vi "PS-RA03B FPGA.vi"() -> ()   [LabVIEW 2011]
uses:
  <vilib>/rvi/eio/common/nirviEmuTemplateMethod_errors.vi
  <vilib>/eio/EIONode/EIONode.xnode
  <vilib>/eio/EIOMethodNode/EIOMethodNode.xnode
  Filter VIs.lvlib
panel:
  out "Timestamp":u32 caption="Tick Count(Ticks)"
  out "Mod5/AI0":fxp<+/-,20,5> format="%.17g"
  out "Mod5/AI2":fxp<+/-,20,5> format="%.17g"
  out "Mod5/AI3":fxp<+/-,20,5> format="%.17g"
  out "Mod1/AI0":fxp<+/-,20,5> format="%.17g"
  out "Mod1/AI1":fxp<+/-,20,5> format="%.17g"
  out "Mod1/AI2":fxp<+/-,20,5> format="%.17g"
  out "Mod1/AI3":fxp<+/-,20,5> format="%.17g"
  out "Mod5/AI1":fxp<+/-,20,5> format="%.17g"
  out "period":u32
  out "delay":u32
  out "dperiod":u32
  out "ACH06-Setpoint":fxp<+/-,20,5>
  out "ALV06B-Setpoint":fxp<+/-,20,5>
  out "ACH05B-Setpoint":fxp<+/-,20,5>
  out "ALV06A-Setpoint":fxp<+/-,20,5>
  out "ACV07A-Setpoint":fxp<+/-,20,5>
  out "ACH07A-Setpoint":fxp<+/-,20,5>
  out "ACV05B-Setpoint":fxp<+/-,20,5>
  out "RRA03B-Setpoint":fxp<+/-,20,5>
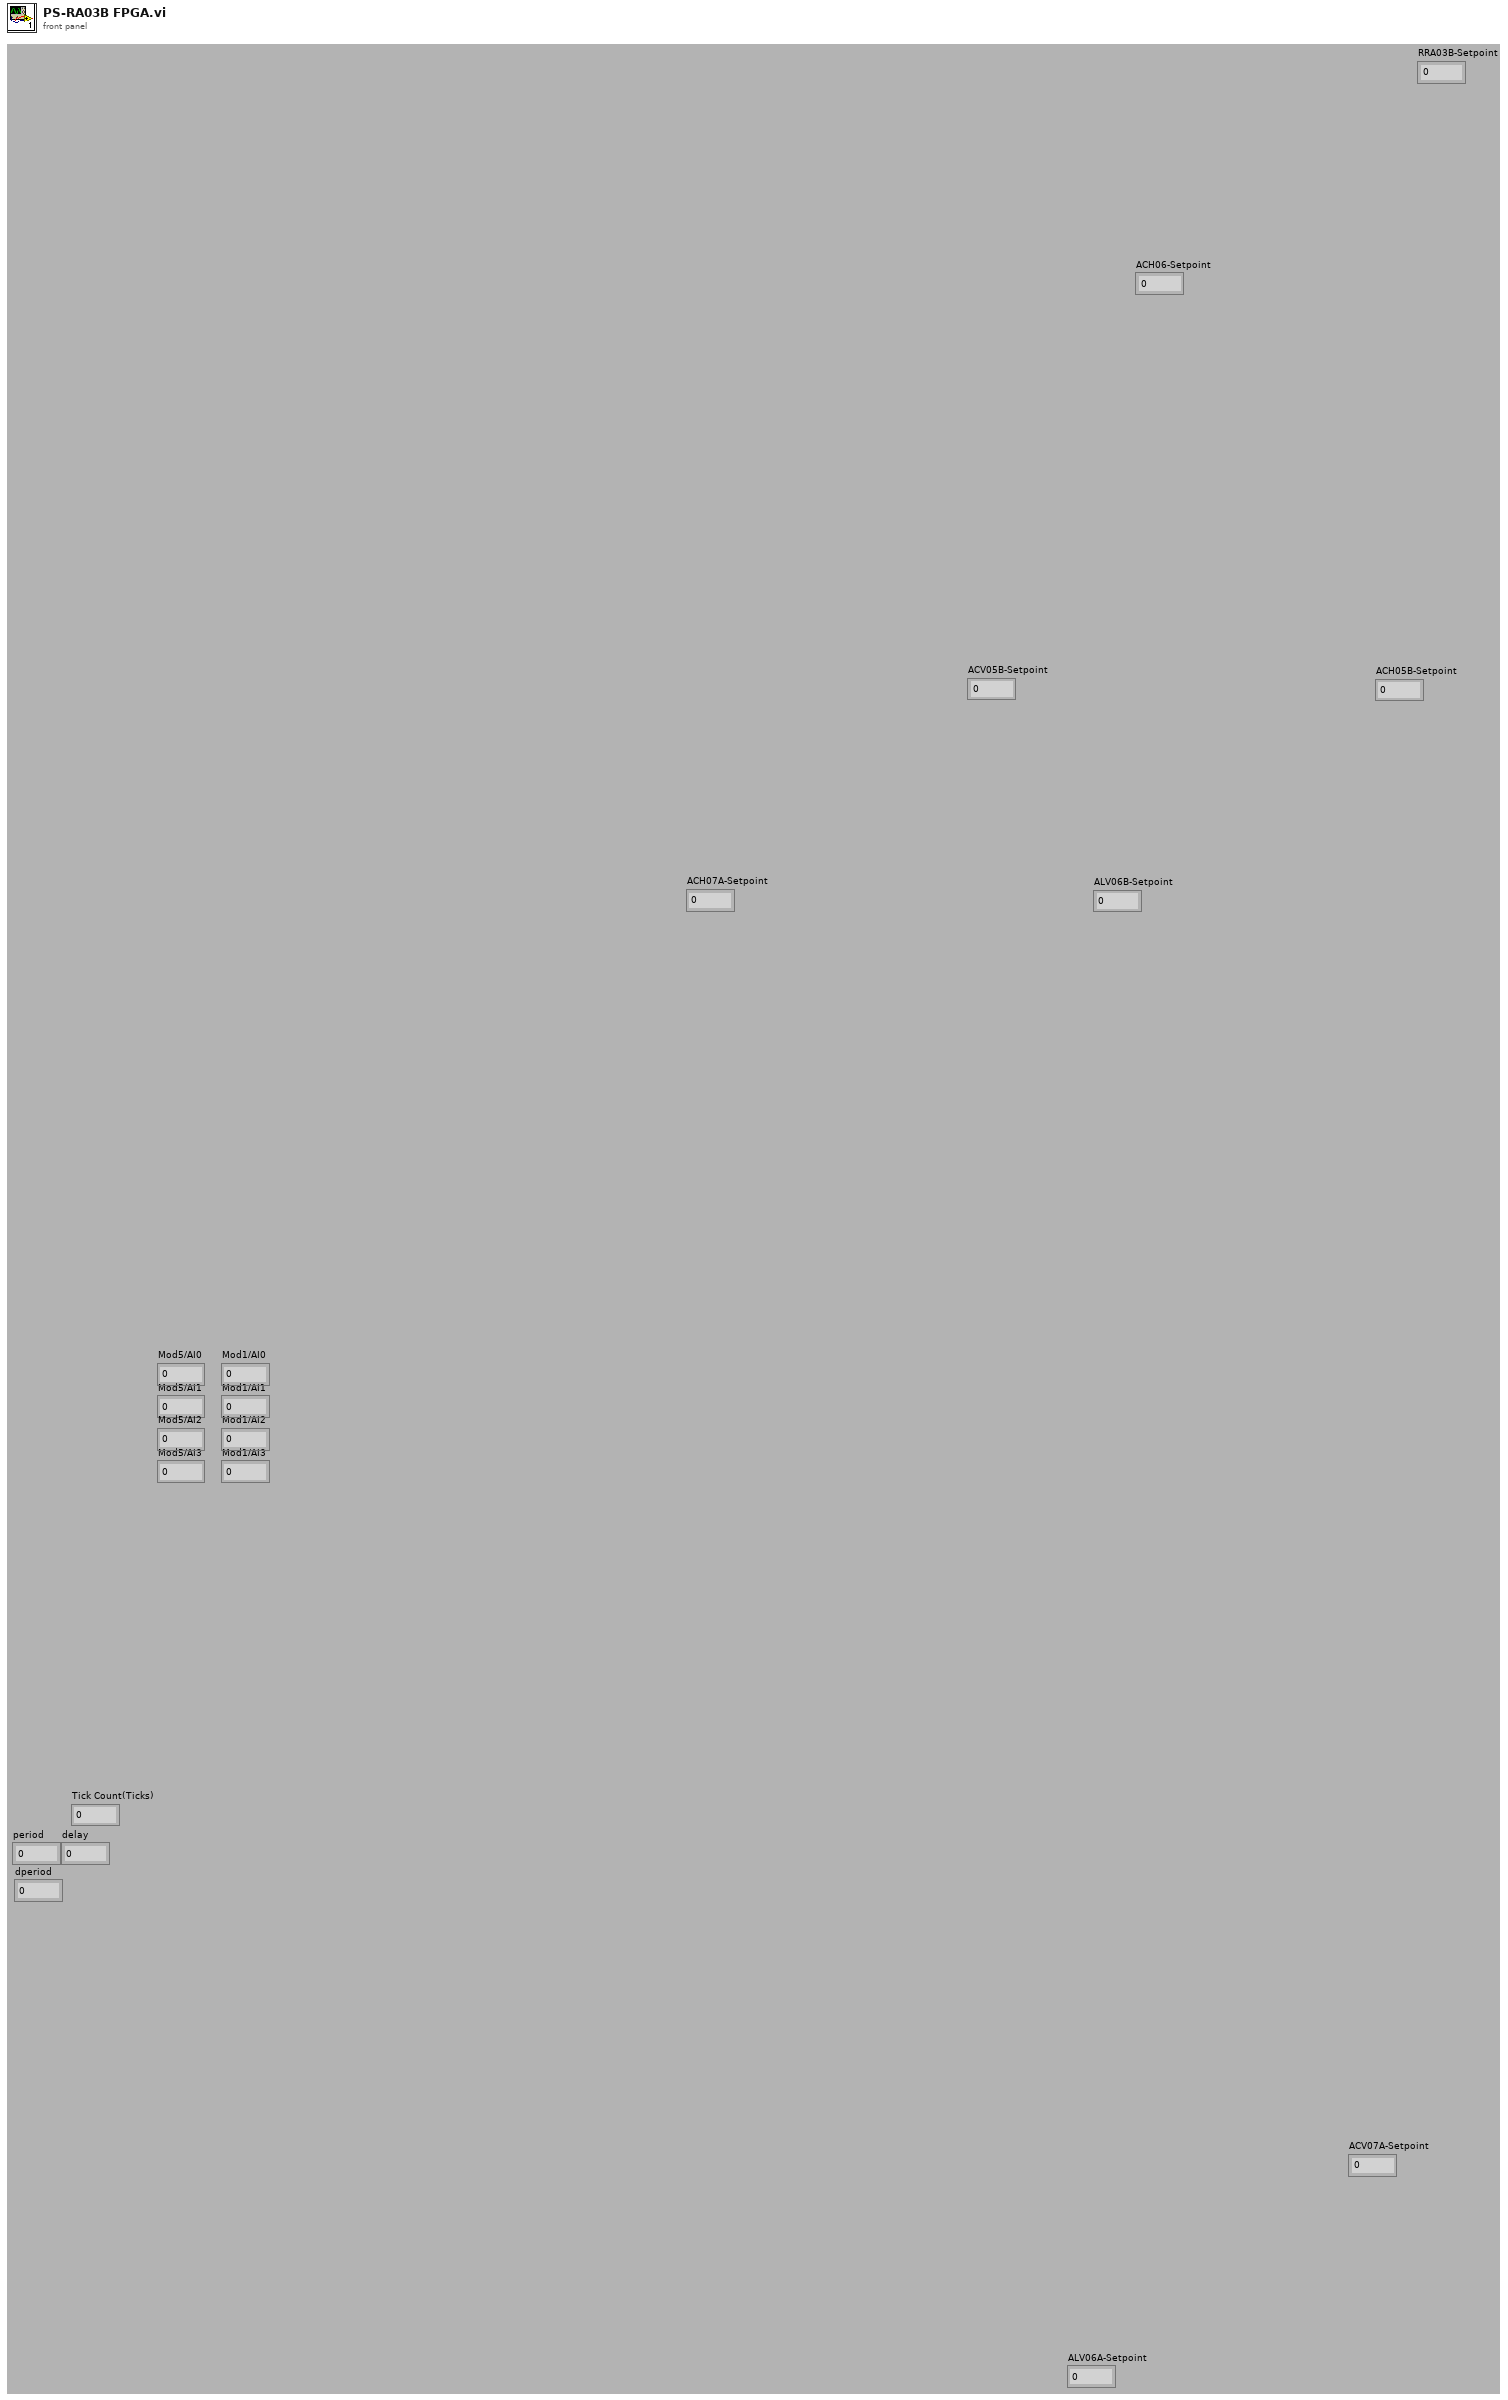
[diagram p1: front panel]
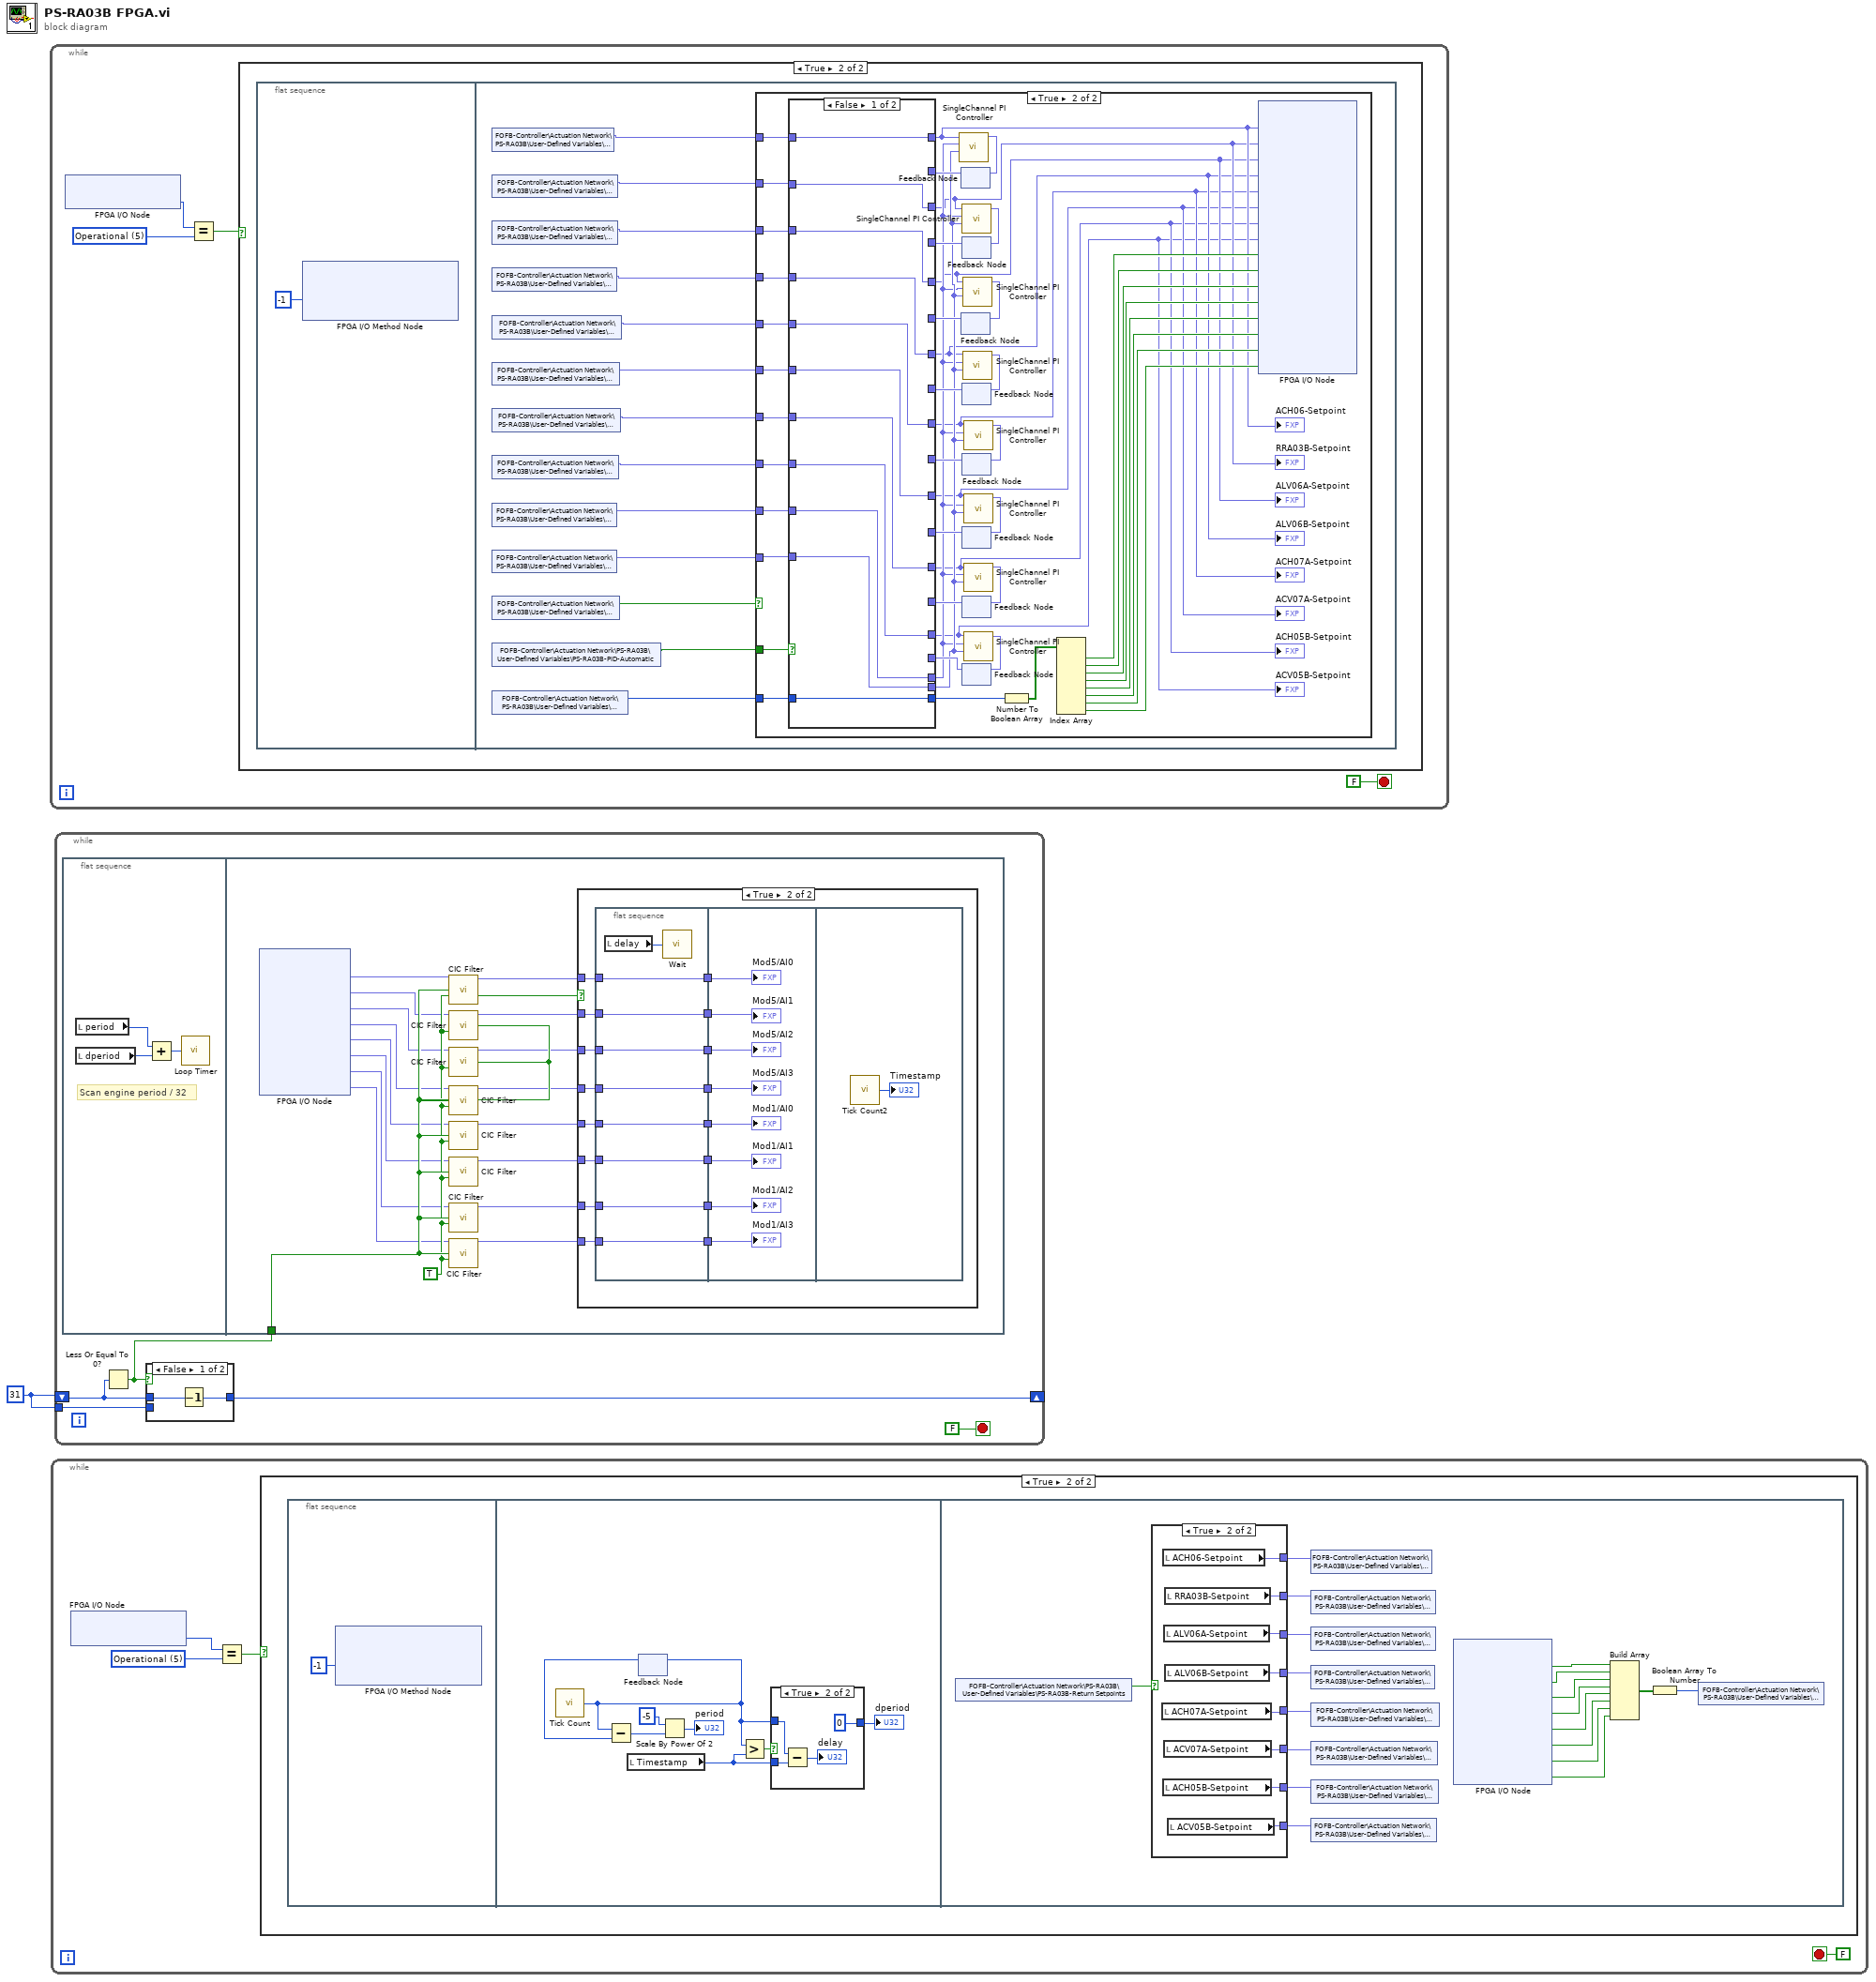
[diagram p0: block diagram]
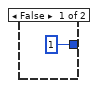
[diagram p5: hidden frame]
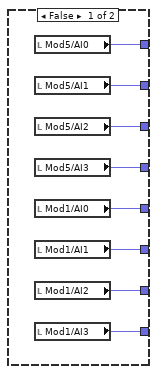
[diagram p6: hidden frame]
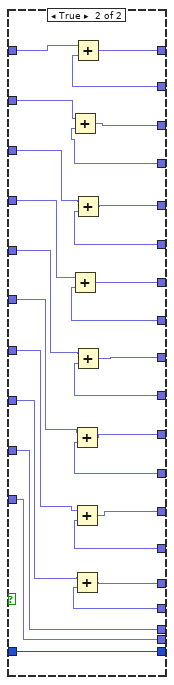
[diagram p9: hidden frame]
diagram:
  w1 = 31
  n1 = while {
    stop <- FALSE stop-if-true
    w4 = u8 5 items=["Init"=1, "PreOp"=2, "Bootstrap"=3, "SafeOp"=4, "Operational"=5]
    n2 = xnode "FPGA I/O Node"() -> ("EtherCAT State"=w3:u8)  [unwired: 1 in, 1 out]
    n3 = Equal?(x=w3, y=w4) -> (x = y?=w2:bool)
    n4 = case shown="True" w2 {
      frame False {
      }
      frame True {
        n5 = flat-sequence {
          frame #0 {
            n6 = xnode "FPGA I/O Method Node"("Timeout"=-1) -> ()  [unwired: 1 in, 2 out]
          }
          frame #1 {
            n7 = shared-variable "FOFB-Controller\\Actuation Network\\PS-RA03B\\User-Defined Variables\\ACH06-Setpoint"() -> (w19:fxp<+/-,20,5>)  [unwired: 1 in, 1 out]
            n8 = shared-variable "FOFB-Controller\\Actuation Network\\PS-RA03B\\User-Defined Variables\\RRA03B-Setpoint"() -> (w18:fxp<+/-,20,5>)  [unwired: 1 in, 1 out]
            n9 = shared-variable "FOFB-Controller\\Actuation Network\\PS-RA03B\\User-Defined Variables\\ALV06A-Setpoint"() -> (w17:fxp<+/-,20,5>)  [unwired: 1 in, 1 out]
            n10 = shared-variable "FOFB-Controller\\Actuation Network\\PS-RA03B\\User-Defined Variables\\ALV06B-Setpoint"() -> (w16:fxp<+/-,20,5>)  [unwired: 1 in, 1 out]
            n11 = shared-variable "FOFB-Controller\\Actuation Network\\PS-RA03B\\User-Defined Variables\\ACH07A-Setpoint"() -> (w15:fxp<+/-,20,5>)  [unwired: 1 in, 1 out]
            n12 = shared-variable "FOFB-Controller\\Actuation Network\\PS-RA03B\\User-Defined Variables\\ACV07A-Setpoint"() -> (w14:fxp<+/-,20,5>)  [unwired: 1 in, 1 out]
            n13 = shared-variable "FOFB-Controller\\Actuation Network\\PS-RA03B\\User-Defined Variables\\ACH05B-Setpoint"() -> (w13:fxp<+/-,20,5>)  [unwired: 1 in, 1 out]
            n14 = shared-variable "FOFB-Controller\\Actuation Network\\PS-RA03B\\User-Defined Variables\\ACV05B-Setpoint"() -> (w12:fxp<+/-,20,5>)  [unwired: 1 in, 1 out]
            n15 = shared-variable "FOFB-Controller\\Actuation Network\\PS-RA03B\\User-Defined Variables\\PS-RA03B-PID-I1"() -> (w11:fxp<+/-,18,1>)  [unwired: 1 in, 1 out]
            n16 = shared-variable "FOFB-Controller\\Actuation Network\\PS-RA03B\\User-Defined Variables\\PS-RA03B-PID-I2"() -> (w10:fxp<+/-,18,2>)  [unwired: 1 in, 1 out]
            n17 = shared-variable "FOFB-Controller\\Actuation Network\\PS-RA03B\\User-Defined Variables\\PS-RA03B-Enable"() -> (w7:bool)  [unwired: 1 in, 1 out]
            n18 = shared-variable "FOFB-Controller\\Actuation Network\\PS-RA03B\\User-Defined Variables\\PS-RA03B-PID-Automatic"() -> (w9:bool)  [unwired: 1 in, 1 out]
            n19 = shared-variable "FOFB-Controller\\Actuation Network\\PS-RA03B\\User-Defined Variables\\PS-RA03B-ON-OFF"() -> (w8:u8)  [unwired: 1 in, 1 out]
            n20 = case shown="True" w7 {
              tunnel: w19 -> [_ w39]
              tunnel: w18 -> [_ w38]
              tunnel: w17 -> [_ w37]
              tunnel: w16 -> [_ w36]
              tunnel: w15 -> [_ w35]
              tunnel: w14 -> [_ w34]
              tunnel: w13 -> [_ w33]
              tunnel: w12 -> [_ w32]
              tunnel: w11 -> [_ w31]
              tunnel: w10 -> [_ w30]
              tunnel: w9 -> [_ w29]
              tunnel: w8 -> [_ w28]
              frame False {
              }
              frame True {
                n21 = feedback #1() -> (w65:fxp<+/-,20,5>)  [unwired: 1 in]
                n22 = feedback #2() -> (w63:fxp<+/-,20,5>)  [unwired: 1 in]
                n23 = feedback #3() -> (w64:fxp<+/-,20,5>)  [unwired: 1 in]
                n24 = feedback #4() -> (w62:fxp<+/-,20,5>)  [unwired: 1 in]
                n25 = feedback #5() -> (w61:fxp<+/-,20,5>)  [unwired: 1 in]
                n26 = feedback #6() -> (w60:fxp<+/-,20,5>)  [unwired: 1 in]
                n27 = feedback #7() -> (w59:fxp<+/-,20,5>)  [unwired: 1 in]
                n28 = feedback #8() -> (w58:fxp<+/-,20,5>)  [unwired: 1 in]
                n29 = case shown="False" w29 {
                  tunnel: w28 -> [w78 w105]
                  tunnel: [w78 w105] -> w66
                  tunnel: [w77 w102] -> w27
                  tunnel: w30 -> [w68 w104]
                  tunnel: [w68 w104] -> w49
                  tunnel: w31 -> [w69 w103]
                  tunnel: [w69 w103] -> w48
                  tunnel: [w76 w97] -> w26
                  tunnel: [w75 w94] -> w25
                  tunnel: [w74 w93] -> w24
                  tunnel: [w73 w92] -> w23
                  tunnel: [w72 w91] -> w22
                  tunnel: [w71 w90] -> w21
                  tunnel: [w70 w89] -> w20
                  tunnel: w65 -> [_ w101]
                  tunnel: w39 -> [w77 w100]
                  tunnel: w64 -> [_ w98]
                  tunnel: w63 -> [_ w95]
                  tunnel: w62 -> [_ w79]
                  tunnel: w61 -> [_ w83]
                  tunnel: w60 -> [_ w86]
                  tunnel: w59 -> [_ w87]
                  tunnel: w58 -> [_ w81]
                  tunnel: w32 -> [w70 w82]
                  tunnel: w33 -> [w71 w88]
                  tunnel: w34 -> [w72 w85]
                  tunnel: w35 -> [w73 w84]
                  tunnel: w36 -> [w74 w80]
                  tunnel: w37 -> [w75 w96]
                  tunnel: w38 -> [w76 w99]
                  frame False {
                  }
                  frame True {
                    n30 = Add(x=w99, y=w98) -> (x+y=w97:fxp<+/-,20,5>)
                    n31 = Add(x=w80, y=w79) -> (x+y=w93:fxp<+/-,20,5>)
                    n32 = Add(x=w85, y=w86) -> (x+y=w91:fxp<+/-,20,5>)
                    n33 = Add(x=w88, y=w87) -> (x+y=w90:fxp<+/-,20,5>)
                    n34 = Add(x=w82, y=w81) -> (x+y=w89:fxp<+/-,20,5>)
                    n35 = Add(x=w100, y=w101) -> (x+y=w102:fxp<+/-,20,5>)
                    n36 = Add(x=w96, y=w95) -> (x+y=w94:fxp<+/-,20,5>)
                    n37 = Add(x=w84, y=w83) -> (x+y=w92:fxp<+/-,20,5>)
                  }
                }
                "ACH06-Setpoint" <- w27
                "ALV06B-Setpoint" <- w24
                "ACH05B-Setpoint" <- w21
                "ALV06A-Setpoint" <- w25
                "ACV07A-Setpoint" <- w22
                "ACH07A-Setpoint" <- w23
                "ACV05B-Setpoint" <- w20
                "RRA03B-Setpoint" <- w26
                n38 = call "SingleChannel PI Controller.vi"("Integral Coefficient a[k]"=w49, "Integral Coefficient b[k]"=w48, "input data"=w27) -> ("output data"=w57:fxp<+/-,20,5>)  [unwired: 8 in]
                n39 = feedback-in #1(w57) -> ()
                n40 = call "SingleChannel PI Controller.vi"("Integral Coefficient a[k]"=w49, "Integral Coefficient b[k]"=w48, "input data"=w26) -> ("output data"=w56:fxp<+/-,20,5>)  [unwired: 8 in]
                n41 = feedback-in #3(w56) -> ()
                n42 = call "SingleChannel PI Controller.vi"("Integral Coefficient a[k]"=w49, "Integral Coefficient b[k]"=w48, "input data"=w25) -> ("output data"=w55:fxp<+/-,20,5>)  [unwired: 8 in]
                n43 = feedback-in #2(w55) -> ()
                n44 = call "SingleChannel PI Controller.vi"("Integral Coefficient a[k]"=w49, "Integral Coefficient b[k]"=w48, "input data"=w24) -> ("output data"=w54:fxp<+/-,20,5>)  [unwired: 8 in]
                n45 = feedback-in #4(w54) -> ()
                n46 = call "SingleChannel PI Controller.vi"("Integral Coefficient a[k]"=w49, "Integral Coefficient b[k]"=w48, "input data"=w23) -> ("output data"=w53:fxp<+/-,20,5>)  [unwired: 8 in]
                n47 = feedback-in #5(w53) -> ()
                n48 = call "SingleChannel PI Controller.vi"("Integral Coefficient a[k]"=w49, "Integral Coefficient b[k]"=w48, "input data"=w22) -> ("output data"=w52:fxp<+/-,20,5>)  [unwired: 8 in]
                n49 = feedback-in #6(w52) -> ()
                n50 = call "SingleChannel PI Controller.vi"("Integral Coefficient a[k]"=w49, "Integral Coefficient b[k]"=w48, "input data"=w21) -> ("output data"=w51:fxp<+/-,20,5>)  [unwired: 8 in]
                n51 = feedback-in #7(w51) -> ()
                n52 = call "SingleChannel PI Controller.vi"("Integral Coefficient a[k]"=w49, "Integral Coefficient b[k]"=w48, "input data"=w20) -> ("output data"=w50:fxp<+/-,20,5>)  [unwired: 8 in]
                n53 = feedback-in #8(w50) -> ()
                n54 = Number To Boolean Array(number=w66) -> (Boolean array=w67:bool[])
                n55 = Index Array(array=w67) -> (element #1=w47:bool, element #2=w46:bool, element #3=w45:bool, element #4=w44:bool, element #5=w43:bool, element #6=w42:bool, element #7=w41:bool, element #8=w40:bool)  [unwired: 8 in]
                n56 = xnode "FPGA I/O Node"("Mod6/AO0"=w27, "Mod6/AO1"=w26, "Mod6/AO2"=w25, "Mod6/AO3"=w24, "Mod2/AO0"=w23, "Mod2/AO1"=w22, "Mod2/AO2"=w21, "Mod2/AO3"=w20, "Mod4/DIO6"=w47, "Mod4/DIO7"=w46, "Mod4/DIO4"=w45, "Mod4/DIO5"=w44, "Mod4/DIO2"=w43, "Mod4/DIO3"=w42, "Mod4/DIO0"=w41, "Mod4/DIO1"=w40) -> ()  [unwired: 16 in, 16 out]
              }
            }
          }
        }
      }
    }
  }
  n57 = while {
    stop <- FALSE stop-if-true
    w108 = u8 5 items=["Init"=1, "PreOp"=2, "Bootstrap"=3, "SafeOp"=4, "Operational"=5]
    n58 = xnode "FPGA I/O Node"() -> ("EtherCAT State"=w107:u8)  [unwired: 1 in, 1 out]
    n59 = Equal?(x=w107, y=w108) -> (x = y?=w106:bool)
    n60 = case shown="True" w106 {
      frame False {
      }
      frame True {
        n61 = flat-sequence {
          frame #0 {
            n62 = xnode "FPGA I/O Method Node"("Timeout"=-1) -> ()  [unwired: 1 in, 2 out]
          }
          frame #1 {
            n63 = call "Tick Count"() -> ("Tick Count(Ticks)"=w112:u32)
            n64 = local read "Timestamp"() -> (w114:u32)
            n65 = feedback #9() -> (w111:u32)  [unwired: 1 in]
            n66 = Subtract(x=w112, y=w111) -> (x-y=w117:u32)
            n67 = feedback-in #9(w112) -> ()
            n68 = Scale By Power Of 2(n=i8 -5, x=w117) -> (x*2^n=→"period":u32)
            n69 = Greater?(x=w112, y=w114) -> (0:w115:bool)
            n70 = case shown="True" w115 {
              tunnel: w112 -> [_ w123]
              tunnel: w114 -> [_ w122]
              tunnel: [u32 1 ("dt 2") u32 0 ("dt 2")] -> w113
              frame False {
              }
              frame True {
                n71 = Subtract(x=w123, y=w122) -> (x-y=→"delay":u32)
              }
            }
            "dperiod" <- w113
          }
          frame #2 {
            n72 = shared-variable "FOFB-Controller\\Actuation Network\\PS-RA03B\\User-Defined Variables\\PS-RA03B-Return Setpoints"() -> (w126:bool)  [unwired: 1 in, 1 out]
            n73 = case shown="True" w126 {
              tunnel: [w150 w158] -> w133
              tunnel: [w149 w157] -> w132
              tunnel: [w148 w155] -> w131
              tunnel: [w147 w156] -> w130
              tunnel: [w146 w154] -> w129
              tunnel: [w145 w153] -> w128
              tunnel: [w144 w152] -> w127
              tunnel: [w143 w151] -> w125
              frame False {
                n74 = local read "Mod5/AI0"() -> (w150:fxp<+/-,20,5>)
                n75 = local read "Mod5/AI1"() -> (w149:fxp<+/-,20,5>)
                n76 = local read "Mod5/AI2"() -> (w148:fxp<+/-,20,5>)
                n77 = local read "Mod5/AI3"() -> (w147:fxp<+/-,20,5>)
                n78 = local read "Mod1/AI0"() -> (w146:fxp<+/-,20,5>)
                n79 = local read "Mod1/AI1"() -> (w145:fxp<+/-,20,5>)
                n80 = local read "Mod1/AI2"() -> (w144:fxp<+/-,20,5>)
                n81 = local read "Mod1/AI3"() -> (w143:fxp<+/-,20,5>)
              }
              frame True {
                n82 = local read "ACH07A-Setpoint"() -> (w154:fxp<+/-,20,5>)
                n83 = local read "ACH06-Setpoint"() -> (w158:fxp<+/-,20,5>)
                n84 = local read "ACH05B-Setpoint"() -> (w152:fxp<+/-,20,5>)
                n85 = local read "ALV06A-Setpoint"() -> (w155:fxp<+/-,20,5>)
                n86 = local read "ACV07A-Setpoint"() -> (w153:fxp<+/-,20,5>)
                n87 = local read "RRA03B-Setpoint"() -> (w157:fxp<+/-,20,5>)
                n88 = local read "ALV06B-Setpoint"() -> (w156:fxp<+/-,20,5>)
                n89 = local read "ACV05B-Setpoint"() -> (w151:fxp<+/-,20,5>)
              }
            }
            n90 = shared-variable "FOFB-Controller\\Actuation Network\\PS-RA03B\\User-Defined Variables\\ACH06-Reading"(w133) -> ()  [unwired: 1 in, 1 out]
            n91 = shared-variable "FOFB-Controller\\Actuation Network\\PS-RA03B\\User-Defined Variables\\RRA03B-Reading"(w132) -> ()  [unwired: 1 in, 1 out]
            n92 = shared-variable "FOFB-Controller\\Actuation Network\\PS-RA03B\\User-Defined Variables\\ALV06A-Reading"(w131) -> ()  [unwired: 1 in, 1 out]
            n93 = shared-variable "FOFB-Controller\\Actuation Network\\PS-RA03B\\User-Defined Variables\\ALV06B-Reading"(w130) -> ()  [unwired: 1 in, 1 out]
            n94 = shared-variable "FOFB-Controller\\Actuation Network\\PS-RA03B\\User-Defined Variables\\ACH07A-Reading"(w129) -> ()  [unwired: 1 in, 1 out]
            n95 = shared-variable "FOFB-Controller\\Actuation Network\\PS-RA03B\\User-Defined Variables\\ACV07A-Reading"(w128) -> ()  [unwired: 1 in, 1 out]
            n96 = shared-variable "FOFB-Controller\\Actuation Network\\PS-RA03B\\User-Defined Variables\\ACH05B-Reading"(w127) -> ()  [unwired: 1 in, 1 out]
            n97 = shared-variable "FOFB-Controller\\Actuation Network\\PS-RA03B\\User-Defined Variables\\ACV05B-Reading"(w125) -> ()  [unwired: 1 in, 1 out]
            n98 = xnode "FPGA I/O Node"() -> ("Mod3/DIO6"=w141:bool, "Mod3/DIO7"=w140:bool, "Mod3/DIO4"=w139:bool, "Mod3/DIO5"=w138:bool, "Mod3/DIO2"=w137:bool, "Mod3/DIO3"=w136:bool, "Mod3/DIO0"=w135:bool, "Mod3/DIO1"=w134:bool)  [unwired: 8 in, 8 out]
            n99 = Build Array(w141, w140, w139, w138, w137, w136, w135, w134) -> (w142:bool[])
            n100 = Boolean Array To Number(Boolean array=w142) -> (number=w124:u8)
            n101 = shared-variable "FOFB-Controller\\Actuation Network\\PS-RA03B\\User-Defined Variables\\PS-RA03B-Status"(w124) -> ()  [unwired: 1 in, 1 out]
          }
        }
      }
    }
  }
  n102 = while {
    shift-right: [w162] -> _
    shift-left: w1 -> [w161]
    tunnel: w1 -> [w159]
    stop <- FALSE stop-if-true
    n103 = flat-sequence {
      tunnel: w160 -> [w188]
      frame #0 {
        # "Scan engine period / 32"
        n104 = local read "period"() -> (w169:u32)
        n105 = local read "dperiod"() -> (w168:u32)
        n106 = Add(x=w169, y=w168) -> (x+y=w167:u32)
        n107 = call "Loop Timer"("Count(Ticks)"=w167) -> ()  [unwired: 1 out]
      }
      frame #1 {
        w187 = TRUE ("input valid")
        n108 = xnode "FPGA I/O Node"() -> ("Mod5/AI0"=w177:fxp<+/-,20,5>, "Mod5/AI1"=w176:fxp<+/-,20,5>, "Mod5/AI2"=w175:fxp<+/-,20,5>, "Mod5/AI3"=w174:fxp<+/-,20,5>, "Mod1/AI0"=w173:fxp<+/-,20,5>, "Mod1/AI1"=w172:fxp<+/-,20,5>, "Mod1/AI2"=w171:fxp<+/-,20,5>, "Mod1/AI3"=w170:fxp<+/-,20,5>)  [unwired: 8 in, 8 out]
        n109 = call "CIC Filter.vi"("input data"=w177, "sample"=w188, "input valid"=w187) -> ("output data"=w185:fxp<+/-,20,5>, "output valid"=w186:bool)  [unwired: 10 in, 1 out]
        n110 = call "CIC Filter.vi"("input data"=w176, "sample"=w188, "input valid"=w187) -> ("output data"=w184:fxp<+/-,20,5>)  [unwired: 10 in, 2 out]
        n111 = call "CIC Filter.vi"("input data"=w175, "sample"=w188, "input valid"=w187) -> ("output data"=w183:fxp<+/-,20,5>)  [unwired: 10 in, 2 out]
        n112 = call "CIC Filter.vi"("input data"=w174, "sample"=w188, "input valid"=w187) -> ("output data"=w182:fxp<+/-,20,5>)  [unwired: 10 in, 2 out]
        n113 = call "CIC Filter.vi"("input data"=w173, "sample"=w188, "input valid"=w187) -> ("output data"=w181:fxp<+/-,20,5>)  [unwired: 10 in, 2 out]
        n114 = call "CIC Filter.vi"("input data"=w172, "sample"=w188, "input valid"=w187) -> ("output data"=w180:fxp<+/-,20,5>)  [unwired: 10 in, 2 out]
        n115 = call "CIC Filter.vi"("input data"=w171, "sample"=w188, "input valid"=w187) -> ("output data"=w179:fxp<+/-,20,5>)  [unwired: 10 in, 2 out]
        n116 = call "CIC Filter.vi"("input data"=w170, "sample"=w188, "input valid"=w187) -> ("output data"=w178:fxp<+/-,20,5>)  [unwired: 10 in, 2 out]
        n117 = case shown="True" w186 {
          tunnel: w185 -> [_ w204]
          tunnel: w184 -> [_ w202]
          tunnel: w183 -> [_ w200]
          tunnel: w182 -> [_ w199]
          tunnel: w181 -> [_ w196]
          tunnel: w180 -> [_ w194]
          tunnel: w179 -> [_ w192]
          tunnel: w178 -> [_ w190]
          frame False {
          }
          frame True {
            n118 = flat-sequence {
              tunnel: w204 -> [w213]
              tunnel: [w213] -> w203
              tunnel: w202 -> [w211]
              tunnel: [w211] -> w201
              tunnel: w200 -> [w209]
              tunnel: w199 -> [w210]
              tunnel: [w210] -> w198
              tunnel: [w209] -> w197
              tunnel: w196 -> [w208]
              tunnel: [w208] -> w195
              tunnel: w194 -> [w207]
              tunnel: [w207] -> w193
              tunnel: w192 -> [w206]
              tunnel: [w206] -> w191
              tunnel: w190 -> [w205]
              tunnel: [w205] -> w189
              tunnel: w203 -> [w220]
              tunnel: w201 -> [w221]
              tunnel: w198 -> [w219]
              tunnel: w197 -> [w218]
              tunnel: w195 -> [w217]
              tunnel: w193 -> [w216]
              tunnel: w191 -> [w215]
              tunnel: w189 -> [w214]
              frame #0 {
                n119 = local read "delay"() -> (w212:u32)
                n120 = call "Wait"("Count(Ticks)"=w212) -> ()  [unwired: 1 out]
              }
              frame #1 {
                "Mod5/AI0" <- w220
                "Mod5/AI2" <- w218
                "Mod5/AI3" <- w219
                "Mod1/AI0" <- w217
                "Mod1/AI1" <- w216
                "Mod1/AI2" <- w215
                "Mod1/AI3" <- w214
                "Mod5/AI1" <- w221
              }
              frame #2 {
                n121 = call "Tick Count2"() -> ("Tick Count(Ticks)"=→"Timestamp":u32)
              }
            }
          }
        }
      }
    }
    n122 = Less Or Equal To 0?(x=w161) -> (x <= 0?=w160:bool)
    n123 = case shown="False" w160 {
      tunnel: [w165 w166] -> w162
      tunnel: w161 -> [w164 _]
      tunnel: w159 -> [_ w166]
      frame False {
        n124 = Decrement(x=w164) -> (x-1=w165:i32)
      }
      frame True {
      }
    }
  }
